vi "Get Variant.vi"(8 "error in (no error)":errorcluster, 9 "Tag":string, 10 "Value Type":refnum<class "Abs_Variant.lvclass">, 11 "Var Bus in":refnum<class "Multi_Bus.lvclass">) -> (0 "error out":errorcluster, 2 "Value Out":refnum<class "Abs_Variant.lvclass">, 3 "Var Bus out":refnum<class "Multi_Bus.lvclass">)   [LabVIEW 2021, in "Multi_Bus.lvclass"]
uses:
  Multi_Bus.lvclass
  Multi_Bus.lvclass/Multi_Bus.ctl
  <vilib>/TSA/Abstract Data Classes/Abs_Types/Variant/Abs_Variant.lvclass
  C:/Program Files (x86)/National Instruments/LabVIEW 2021/vi.lib/TSA/Abstract Data Classes/Abs_Types/Value/Abs_Value.lvclass
  C:/Program Files (x86)/National Instruments/LabVIEW 2021/vi.lib/TSA/Abstract Data Classes/Abs_Types/Type/Abs_Type.lvclass
  C:/Program Files (x86)/National Instruments/LabVIEW 2021/vi.lib/TSA/Abstract Data Classes/Abs_Types/Variant/Abs_Variant.lvclass
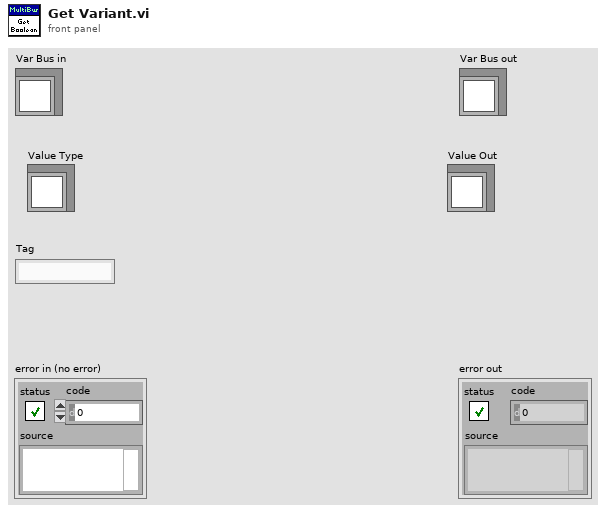
[diagram p1: front panel]
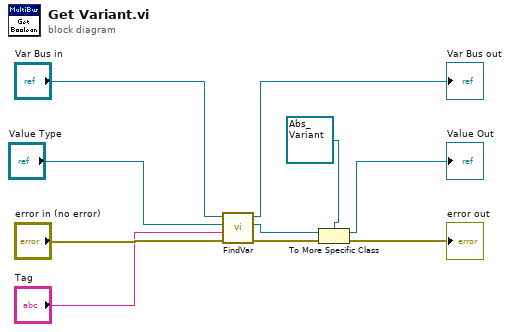
[diagram p0: block diagram]
diagram:
  n1 = call "FindVar.vi"("error in (no error)"="error in (no error)", "Tag"="Tag", "Abs_Type Default"="Value Type", "Var Bus in"="Var Bus in") -> ("error out"=w7:errorcluster, "Abs_Type Found"=w6:refnum<class "Abs_Type.lvclass">, "Var Bus out"=→"Var Bus out":refnum<class "Multi_Bus.lvclass">)  [unwired: 5 in]
  n2 = To More Specific Class(target class=refnum<class "Abs_Variant.lvclass"> refnum ("Abs_U8 Integer.lvclass Out"), reference=w6, error in=w7) -> (specific class reference=→"Value Out":refnum<class "Abs_Variant.lvclass">, error out=→"error out":errorcluster)
